vi "Circular.vi"() -> ()   [LabVIEW 2018]
uses:
  D:/CircularWPF/LV-Source/CircularWF.dll
  CircularWF.dll
panel:
  in  "Horizontal Pointer Slide":dbl(slide)=36.592178770949715 scale=0.0..100.0
  in  "Stop Button":bool
  in  "CircularWF":refnum<k24>(container)
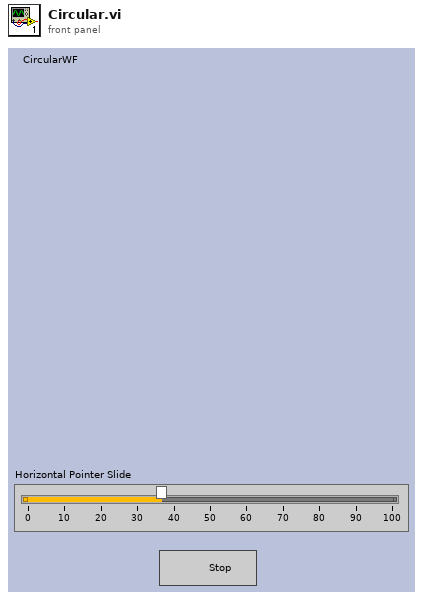
[diagram p1: front panel]
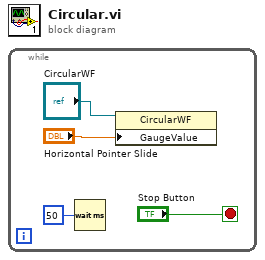
[diagram p0: block diagram]
diagram:
  n1 = while {
    stop <- "Stop Button" stop-if-true
    n2 = Wait (ms)(milliseconds to wait=u32 50) -> ()  [unwired: 1 out]
    n3 = property class="CircularWF"(reference="CircularWF", "GaugeValue"="Horizontal Pointer Slide") -> ()  [unwired: 1 in, 2 out]
  }
